vi "Finish.vi"(8 "error in (no error)":errorcluster, 10 "Warnings":string[](array[string]), 11 "SaveForPrevious in":refnum<class "SaveForPrevious.lvclass">) -> (0 "error out":errorcluster, 1 "Output/Failure":string, 3 "SaveForPrevious out":refnum<class "SaveForPrevious.lvclass">)   [LabVIEW 2014, in "SaveForPrevious.lvclass"]
doc: "Processes warnings and sets output message for the operation."
uses:
  SaveForPrevious.lvclass
  SaveForPrevious.lvclass/SaveForPrevious.ctl
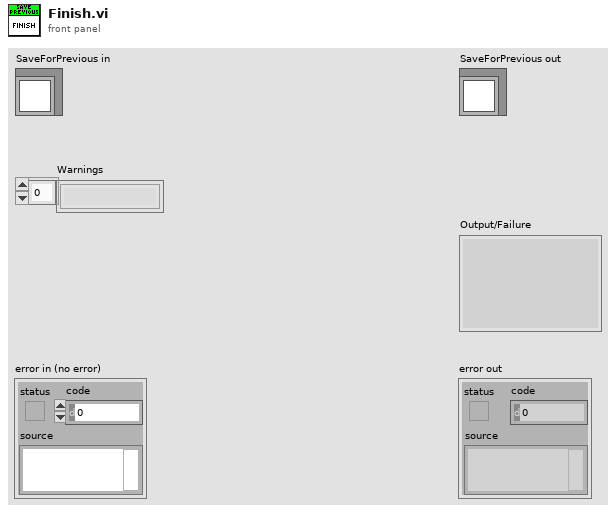
[diagram p1: front panel]
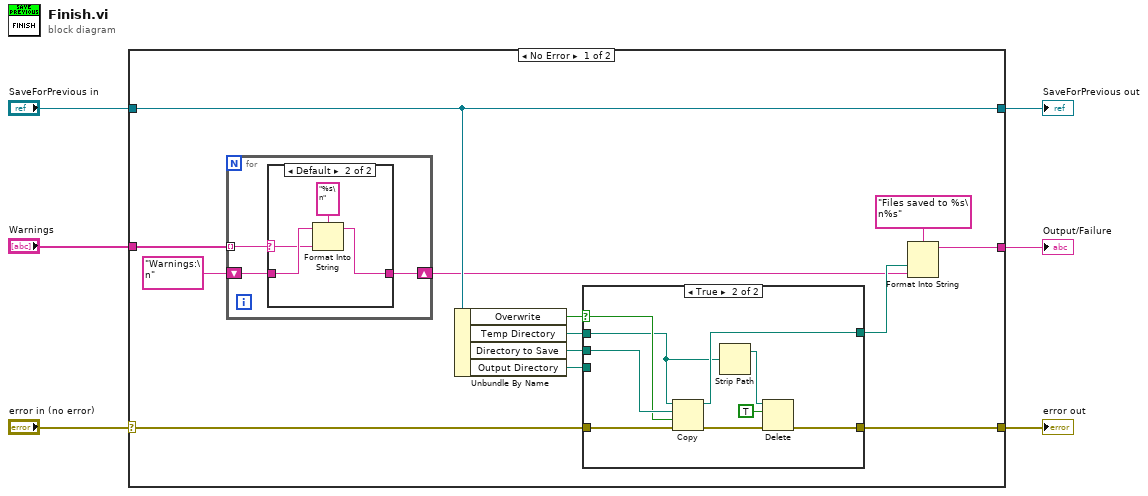
[diagram p0: block diagram]
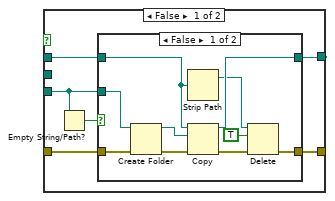
[diagram p3: hidden frame]
diagram:
  n1 = case shown="No Error" "error in (no error)" {
    selector: "error in (no error)" -> [w8 w56]
    tunnel: [w7 w56] -> w5
    tunnel: [w18 w55] -> w3
    tunnel: "SaveForPrevious in" -> [w18 w55]
    tunnel: "Warnings" -> [w19 _]
    tunnel: [w10 _] -> w1
    frame No Error {
      n2 = for {
        tunnel: w19 -> [w20] mode=indexing
        shift-right: [w21] -> w11
        shift-left: "Warnings:\n" -> [w22]
        n3 = case shown="Default" w20 {
          selector: w20 -> [_ w24]
          tunnel: w22 -> [w23 w27]
          tunnel: [w23 w26] -> w21
          frame "" {
          }
          frame Default {
            n4 = Format Into String(format string="%s\n", initial string=w27, w24) -> (resulting string=w26:string)  [unwired: 1 in, 1 out]
          }
        }
      }
      n5 = Unbundle By Name(w18) -> ("Overwrite"=w17:bool, "Temp Directory"=w16:path, "Directory to Save"=w15:path, "Output Directory"=w14:path)
      n6 = case shown="True" w17 {
        selector: w17 -> [_ w53]
        tunnel: w16 -> [w31 w51]
        tunnel: w15 -> [_ w54]
        tunnel: w14 -> [w32 _]
        tunnel: [w30 w52] -> w12
        tunnel: w8 -> [w29 w50]
        tunnel: [w28 w49] -> w7
        frame False {
          n7 = Empty String/Path?(string/path=w32) -> (empty?=w33:bool)
          n8 = case shown="False" w33 {
            tunnel: w32 -> [w43 _]
            tunnel: w31 -> [w35 w45]
            tunnel: [w42 w45] -> w30
            tunnel: w29 -> [w41 w44]
            tunnel: [w40 w44] -> w28
            frame False {
              n9 = Create Folder(path (use dialog)=w43, error in=w41) -> (created path=w39:path, error out=w37:errorcluster)  [unwired: 1 in, 1 out]
              n10 = Strip Path(path=w35) -> (stripped path=w34:path)  [unwired: 1 out]
              n11 = Copy(8:w37, 10:w39, 11:w35) -> (0:w36:errorcluster, 3:w42:path)  [unwired: 2 in, 1 out]
              n12 = Delete(path (use dialog)=w34, entire hierarchy (F)=TRUE, error in=w36) -> (error out=w40:errorcluster)  [unwired: 2 in, 2 out]
            }
            frame True {
            }
          }
        }
        frame True {
          n13 = Copy(8:w50, 9:w53, 10:w54, 11:w51) -> (0:w48:errorcluster, 3:w52:path)  [unwired: 1 in, 1 out]
          n14 = Strip Path(path=w51) -> (stripped path=w46:path)  [unwired: 1 out]
          n15 = Delete(path (use dialog)=w46, entire hierarchy (F)=TRUE, error in=w48) -> (error out=w49:errorcluster)  [unwired: 2 in, 2 out]
        }
      }
      n16 = Format Into String(format string="Files saved to %s\n%s", w12, w11) -> (resulting string=w10:string)  [unwired: 2 in, 1 out]
    }
    frame Error {
    }
  }
  "error out" <- w5
  "SaveForPrevious out" <- w3
  "Output/Failure" <- w1
